vi "viewer.vi"(8 "Color Box":u32(colorbox)=5896447, 11 "Ibeo":dbl[][](array[numeric])=[[-8.194514690670069, 12.209047268904888, 0.20057577918921865, -1.2], [-7.922188195282239, 12.530063176191208, 0.1993192339962172, -1.2], [-7.848906696184014, 12.605199714224918, 0.19910980979738363, -1.2], [-8.31093082702301, 12.33609318816849, 0.3656663756006245, -0.3999999999999999], [-8.273047603432309, 12.451558326925204, 0.36524749998274675, -0.3999999999999999], [-8.066578783002836, 12.699122833174604, 0.36489843696784874, -0.3999999999999999], [-7.908452357315748, 12.841755311057485, 0.1945024774230451, -1.2], [-7.895234983174988, 12.994568657418597, 0.19219881123587584, -1.2], [-8.062522647946755, 12.859777292173597, 0.3640606857320933, -0.3999999999999999], [-7.824791817030648, 13.99344470034109, 0.17649199632335816, -1.2], [-8.063674699079533, 13.931801029401951, 0.3581964270818056, -0.3999999999999999], [-7.8135978930264125, 14.173967995680819, 0.17356005753968817, -1.2], [-8.031209860249872, 14.080843843301425, 0.35749830105200947, -0.3999999999999999], [-7.82276958407434, 14.387850587687291, 0.1697904219606839, -1.2], [-8.073152114569078, 14.335283323635828, 0.3558926111834783, -0.3999999999999999], [-7.891075140636294, 14.693334221257622, 0.1637171201945104, -1.2], [-8.111243508180511, 14.591251758204468, 0.35428692131494716, -0.3999999999999999], [-7.837216119361166, 14.82676657508684, 0.16204172660384186, -1.2], [-8.065161930030882, 14.734022733414673, 0.35365860788813064, -0.3999999999999999], [-7.8864594284729, 15.11851517851068, 0.15638727323533547, -1.2], [-8.136133319461743, 15.049896083998677, 0.35156422979874213, -0.3999999999999999], [-8.062386760128094, 15.160595778342891, 0.35121516678384407, -0.3999999999999999], [-7.9015329362479765, 15.597469450579638, 0.14780088108315914, -1.2], [-8.030734784039595, 15.565267383057458, 0.3489811634884964, -0.3999999999999999], [-7.837442171074448, 15.732479146376736, 0.14612548749249055, -1.2], [-8.048111766595339, 15.827552126486646, 0.34737547361996524, -0.3999999999999999], [-7.860387428879935, 16.012208734234335, 0.1408898825216513, -1.2], [-8.056202749080104, 16.08256925295217, 0.3458395963544137, -0.3999999999999999], [-7.87387677823714, 16.284689646223693, 0.13586370174964563, -1.2], [-7.837519828869938, 16.480818892560503, 0.13272233876714212, -1.2], [-8.06566035168659, 16.347183699638233, 0.3442339064858825, -0.3999999999999999], [-11.669869640901991, 13.268898159351348, 0.3442339064858825, -0.3999999999999999], [-11.623722029161186, 13.581091757690992, 0.34304709223522906, -0.3999999999999999], [-7.823316745669438, 16.72057446606854, 0.12853385479047075, -1.2], [-8.055641790260522, 16.587197426343405, 0.3428376544262902, -0.3999999999999999], [-8.042029216167052, 16.82800693693079, 0.3414414023666979, -0.3999999999999999], [-7.820276479008444, 16.98716777957602, 0.1237170982172986, -1.2], [-11.673363951247808, 13.989217618076957, 0.34088290154286094, -0.3999999999999999], [-11.802226900015416, 13.921712225849964, 0.34053383852796293, -0.3999999999999999], [-8.049807482572618, 17.112867929828568, 0.3396960872922075, -0.3999999999999999], [-11.712420247707064, 14.212131313250396, 0.3396262746892279, -0.3999999999999999], [-11.712185704759628, 14.402104547594199, 0.3387187108504929, -0.3999999999999999], [-11.680735996678221, 14.56510231725602, 0.33809039742367636, -0.3999999999999999], [-7.8114890300212805, 17.540707439157913, 0.1136647366732873, -1.2], [-8.018268387774892, 17.624731922838397, 0.33669414536408404, -0.3999999999999999], [-11.72577268948283, 14.805480140404125, 0.33669414536408404, -0.3999999999999999], [-7.800708178599534, 17.818889350133773, 0.10863855590128157, -1.2], [-11.710914134211848, 14.990914134211849, 0.33585639412832863, -0.3999999999999999], [-11.665658577131227, 15.1484193030316, 0.3352978933044917, -0.3999999999999999], [-8.027699153236274, 17.938916949360994, 0.33473939248065476, -0.3999999999999999], [-7.804112965736486, 18.133414204998054, 0.1027746783339416, -1.2], [-8.011648084453142, 18.061238599938417, 0.5659587335491414, 0.40000000000000013], [-8.014847599185678, 18.067193186426245, 0.7980630184613928, 1.2000000000000006], [-11.701887182530728, 15.392329358999303, 0.3339016412448994, -0.3999999999999999], [-11.18235494553231, 15.899808863285491, 0.3337620160389402, -0.3999999999999999], [-8.0322354499762, 18.254328816861292, 0.3327846395972256, -0.3999999999999999], [-11.62775268829881, 15.738382844333326, 0.3325053891853071, -0.3999999999999999], [-11.73472519046489, 15.637753162553611, 0.3325053891853071, -0.3999999999999999], [-7.802601115554845, 18.449075343828376, 0.09691080076660175, -1.2], [-8.008769879914695, 18.526556479295465, 0.33117894972869444, -0.3999999999999999], [-7.831841217452702, 18.837389870324824, 0.08937152960859324, -1.2], [-7.985685070733222, 18.808397837650894, 0.3295034472571836, -0.3999999999999999], [-7.762836832549808, 19.038628603093233, 0.08623016662608962, -1.2], [-7.998428267279901, 19.17151180169247, 0.3271996313588563, -0.3999999999999999], [-7.807112712480842, 19.4834706448484, 0.07743435027507978, -1.2], [-8.036104747242254, 19.598910858367518, 0.3244071272396717, -0.3999999999999999], [-8.021956225472685, 19.750254373746202, 0.5765004365990634, 0.40000000000000013], [-8.049686111962624, 19.992036352840987, 0.3218938735324055, -0.3999999999999999], [-7.994407959440638, 20.062524792131466, 0.578385376879513, 0.40000000000000013], [-8.040090666069212, 20.350354036833295, 0.3196598702370579, -0.3999999999999999], [-7.999678783030214, 20.45726955656002, 0.5808986305867792, 0.40000000000000013], [-8.024832769245576, 20.7097434285252, 0.31742586694171016, -0.3999999999999999], [-7.9904318259420295, 20.835113251217667, 0.5832722590880861, 0.40000000000000013], [-8.0201622485404, 21.106673826814433, 0.31491261323444397, -0.3999999999999999], [-7.995314329012896, 21.25983310220247, 0.5859949506042911, 0.40000000000000013], [-8.001177834809809, 21.48647283041383, 0.31253898473313707, -0.3999999999999999], [-7.9575040474444485, 22.048783880339585, 0.5909516454158438, 0.40000000000000013], [-8.046483670341773, 22.0329497364633, 0.308908729378197, -0.3999999999999999], [-8.025433114646795, 22.442977434942478, 0.3063256630679513, -0.3999999999999999], [-7.9802625842223485, 22.569711190455976, 0.594372462961845, 0.40000000000000013], [-8.009054805576646, 22.88184322956092, 0.30353315894876665, -0.3999999999999999], [-7.968571393744589, 23.027403979048092, 0.5973045922869888, 0.40000000000000013], [-7.990899654200996, 23.856241946520424, 0.2972500246806013, -0.3999999999999999], [-8.000898076518773, 24.152091251589102, 0.6047047282028281, 0.40000000000000013], [-8.011964114086332, 24.457778204016666, 0.29327070631076324, -0.3999999999999999], [-7.972054867346523, 24.63260748666816, 0.6077764827339311, 0.40000000000000013], [-7.988910651645925, 24.9672300085195, 0.28998951397072126, -0.3999999999999999], [-7.938790538019864, 25.123578481570966, 0.6109180498680138, 0.40000000000000013], [-7.984256066269928, 25.553256654635888, 0.2861498208068424, -0.3999999999999999], [-7.943696922487425, 25.74772056172415, 0.6150369934438111, 0.40000000000000013], [-8.005768122858095, 26.24480723490346, 0.2815421890101878, -0.3999999999999999], [-7.973645924100258, 26.477717681601202, 0.6199238756523843, 0.40000000000000013], [-7.996752928404116, 26.88147248348014, 0.2773534328314109, -0.3999999999999999], [-7.966378125571135, 27.133912528293944, 0.6242522570371204, 0.40000000000000013], [19.072594357887944, 19.847646565571097, 0.273513739667532, -0.3999999999999999], [-7.974119624650943, 27.510164161678034, 0.27323448925561356, -0.3999999999999999], [18.966327804266037, 20.047570235996055, 0.2731646766526339, -0.3999999999999999], [18.940416091600433, 20.31977342712424, 0.2720476750049601, -0.3999999999999999], [-7.966530139110388, 27.848833218611254, 0.6289995140397342, 0.40000000000000013], [19.617239241951573, 20.16420326208543, 0.6308146417172042, 0.40000000000000013], [19.470454947247852, 20.336065589851415, 0.6308146417172042, 0.40000000000000013], [-7.938090412265838, 28.130667071877102, 0.26918535828279583, -0.3999999999999999], [19.481777877437366, 20.34582205069638, 0.9928275233766126, 1.2000000000000006], [19.68969208752365, 20.225539123400168, 0.9945029169672812, 1.2000000000000006], [-7.904373212400746, 28.403162954359185, 0.6325599567916946, 0.40000000000000013], [-11.218347998608445, 29.1922777087403, 0.645754538754842, 0.40000000000000013], [-11.255655930488722, 29.279114272061154, 1.0393196955176651, 1.2000000000000006], [-7.931052931321677, 30.565756380981856, 0.2529190217885454, -0.3999999999999999], [-7.915722020860143, 30.965173285836535, 0.64973385712468, 0.40000000000000013], [19.643079014175772, 25.999680999909852, 0.6595774341448059, 0.40000000000000013], [19.678772386784143, 26.04038149087464, 1.0799479900913775, 1.2000000000000006], [19.794377409040397, 25.97301782491852, 0.23986406503135732, -0.3999999999999999], [16.951716843249166, 28.313152412727153, -0.18246108047738013, -1.2], [17.23702345210269, 28.261242886298856, -0.18497417086338291, -1.2], [17.355126239459604, 28.42991114665332, 0.2369319357062135, -0.3999999999999999], [17.500999358199543, 28.40558641198749, 1.0906286242318897, 1.2000000000000006], [17.521755060239993, 28.434955051084508, 0.6637661903235827, 0.40000000000000013], [-9.551271036081815, 33.70704072673605, 1.1140841345012495, 1.2000000000000006], [17.026214692366207, 30.91768945041584, -0.22895325261843263, -1.2], [16.947627408349614, 31.330792132214754, -0.23544540278227327, -1.2], [21.974210360871428, 29.796607180878567, 0.20970502054416343, -0.3999999999999999], [21.858954092414884, 29.892890962266808, 0.6902949794558367, 0.40000000000000013], [23.61693994019074, 29.825860936769622, 0.2020256342164057, -0.3999999999999999], [26.517784402942883, 29.636358746131258, 0.18897067745921764, -0.3999999999999999], [26.28807825554624, 29.868078255546244, 0.18897067745921764, -0.3999999999999999], [27.494195142074055, 29.89355973078797, 0.7171728316029887, 0.40000000000000013], [-9.596819805221863, 41.319124757332645, 0.17738178536460142, -0.3999999999999999], [-9.614421585529625, 42.10789864388739, 0.727993785064829, 0.40000000000000013], [-9.657997961001028, 43.03366172097774, 0.16565326806402603, -0.3999999999999999], [-9.654708582864293, 43.79505415648642, 0.7395128645564657, 0.40000000000000013], [-9.644952612918221, 44.55715817032658, 0.15532100282304295, -0.3999999999999999], [-9.649848604658922, 44.578365040432125, -0.43460781587299796, -1.2], [-9.613637000791527, 45.25325758295734, 1.3482203887971804, 1.2000000000000006], [-9.659620726679865, 45.4564764101684, 0.7508225062391634, 0.40000000000000013], [-9.631988411628107, 46.20048575995598, 0.14415098634630447, -0.3999999999999999], [-9.607672332879817, 47.92485002284773, 0.13242246904572907, -0.3999999999999999], [17.086090559334245, 45.56061718044098, 1.4035083772892427, 1.2000000000000006], [17.292711367504157, 45.540430347987886, -0.5047649224822437, -1.2], [17.52268129512945, 45.574561388711366, 1.407278012868247, 1.2000000000000006], [17.557063414189265, 45.656553436391754, 0.7696719090436596, 0.40000000000000013], [15.905718653071306, 48.76995079198919, 0.11420137966804939, -0.3999999999999999], [15.711030412050338, 48.84901591474403, 0.7858684329349304, 0.40000000000000013], [27.308705200532295, 43.3826639824295, 0.11154850075482398, -0.3999999999999999], [27.522668444206523, 43.31998672256406, 0.7889401874660336, 0.40000000000000013], [25.383882599796944, 45.09750939942709, 0.10882580923861901, -0.3999999999999999], [15.378656492958747, 49.840262152105595, -0.5751314532903231, -1.2], [15.600149970456558, 49.82844562031466, 0.7920817546001162, 0.40000000000000013], [15.416587087242455, 49.95362474886922, 0.1074993697820063, -0.3999999999999999], [25.68368027358097, 46.42446403292412, 0.09981998345424858, -0.3999999999999999], [25.383632788769415, 46.777506687909195, 0.09877279440955439, -0.3999999999999999], [-8.027847677156654, 53.1687727040271, 0.09842373139465632, -0.3999999999999999], [-8.695167719437398, 53.15994682681221, 0.80227439463514, 0.40000000000000013], [20.483247073305144, 49.77303169169489, 0.09584066508441053, -0.3999999999999999], [20.078047311320553, 49.95132385408298, 0.09584066508441053, -0.3999999999999999], [19.718193698014808, 50.23653112811276, 0.09500291384865517, -0.3999999999999999], [25.429376633443997, 47.73477995506515, 0.09283872315628705, -0.3999999999999999], [-9.338780758706811, 54.24462327975186, 0.8105122817867347, 0.40000000000000013], [16.860460258517662, 52.83196371705928, -0.6444508631042345, -1.2], [25.652365748645803, 49.03552706564198, 0.08418196038681475, -0.3999999999999999], [32.06392885145435, 45.03486562995687, 1.5521995584610773, 1.2000000000000006], [31.778479775771135, 45.41808238881591, 0.818261480717472, 0.40000000000000013], [31.77225525537603, 45.40989672895938, 1.55471264884708, 1.2000000000000006], [25.423084254782847, 49.565065245207975, 0.08173851928252823, -0.3999999999999999], [32.6300247772637, 45.011263200800904, 1.559110557022585, 1.2000000000000006], [32.69832444037635, 45.09790091043385, 0.8204256714098401, 0.40000000000000013], [25.439400701881368, 50.55981320376924, 0.075595010220322, -0.3999999999999999], [34.51917188715493, 45.11514830598214, 1.5857074302744485, 1.2000000000000006], [34.92683747694728, 44.86443385971285, 1.5871733996662833, 1.2000000000000006], [25.42149285051838, 51.52298336238443, 0.06973075157003433, -0.3999999999999999], [35.54812755297423, 44.85971643116604, 1.595550367619626, 1.2000000000000006], [34.609532792271075, 45.973543243462, 1.6007859725904654, 1.2000000000000006], [25.46718877424603, 52.64016177857301, 0.06267967866909313, -0.3999999999999999], [34.731322610921104, 46.89122723132968, 1.6173304842983174, 1.2000000000000006], [25.468059591047258, 53.70827288404634, 0.05604748138602972, -0.3999999999999999], [41.47455368343372, 42.586470182247886, 1.6470687205326844, 1.2000000000000006], [25.474515940300442, 54.8248279005798, 0.04906622108806813, -0.3999999999999999], [17.65203521232784, 58.21903070119556, 0.04780959423443509, -0.3999999999999999], [20.295637544941265, 57.39533782171512, 0.8528885317953614, 0.40000000000000013], [17.443289950392376, 58.39142219368391, 0.8528885317953614, 0.40000000000000013], [20.330615094364084, 57.487659485279245, 1.6608907176556997, 1.2000000000000006], [-7.75035495317097, 61.16042739371937, 0.04348121284969886, -0.3999999999999999], [17.389741843531517, 59.058954065737105, 0.04278308681990278, -0.3999999999999999], [25.459018306497637, 55.93626861288663, 0.04215477339308621, -0.3999999999999999], [43.67980265747188, 42.54959453739267, 0.8601490425052414, 0.40000000000000013], [43.68617582564682, 42.555282807469325, 1.680786016544889, 1.2000000000000006], [35.131445440240526, 50.67758542316679, 1.685183924720394, 1.2000000000000006], [25.54658114567024, 57.304002719404814, 0.033288572814675066, -0.3999999999999999], [35.35626866103595, 51.854440322607054, 1.7078017381944195, 1.2000000000000006], [31.93987374886766, 54.289371727955974, 1.7096865559839216, 1.2000000000000006], [32.39423109821591, 54.025674009004575, 0.8699926195253671, 0.40000000000000013], [31.951466968313056, 54.30774586871799, 0.8699926195253671, 0.40000000000000013], [32.40411221068225, 54.04103591888299, 1.710524252779256, 1.2000000000000006], [17.757709303896025, 61.10224897949335, 0.8715983093938983, 0.40000000000000013], [17.763112456640282, 61.11964997506754, 1.715341009352428, 1.2000000000000006], [35.4230011788845, 52.84401581410436, 1.7253933708964393, 1.2000000000000006], [29.290605081293037, 57.09313695219341, 0.8773229428382268, 0.40000000000000013], [40.759454288225115, 49.265171081946534, 1.7369117018322857, 1.2000000000000006], [40.82070045763014, 49.33379161726375, 0.8795569461335744, 0.40000000000000013], [30.505508525730225, 57.06601565541906, 0.8813022612080648, 0.40000000000000013], [41.460377534907316, 49.23945311745191, 1.7463357907797963, 1.2000000000000006], [31.138639213649242, 57.081515746789364, 0.8836060771063922, 0.40000000000000013], [46.014679894453145, 45.363042821123074, 1.7563881523238076, 1.2000000000000006], [31.743685463928472, 57.03846551713426, 0.8854910173868418, 0.40000000000000013], [17.31309627006752, 63.34316908027608, 1.757225849119142, 1.2000000000000006], [42.29288815694243, 49.34445773182582, 1.7597389395051446, 1.2000000000000006], [42.32831546364073, 49.38278277629349, 0.886887269446434, 0.40000000000000013], [17.88136701557938, 63.34167325680246, 1.760576636300479, 1.2000000000000006], [17.62830080143847, 63.44853765546489, -0.8612049088969791, -1.2], [26.330614951038932, 60.21786202185187, 0.012554229729729194, -0.3999999999999999], [17.65164798186575, 63.527356415664414, 0.012414604523770023, -0.3999999999999999], [47.01008426653839, 44.78828389450921, 1.763927423481816, 1.2000000000000006], [32.40222865539054, 57.07441257637522, 0.8880740836970875, 0.40000000000000013], [25.875513670239723, 60.537777650039054, 0.011856103699933118, -0.3999999999999999], [26.6293328816576, 60.21031030179518, 0.8882835215060264, 0.40000000000000013], [46.08014715978688, 46.16470846246666, 1.7687441800549881, 1.2000000000000006], [42.986510275999805, 49.28546090702975, 1.7687441800549881, 1.2000000000000006], [43.001773126855184, 49.30168579532624, 0.8896797735656188, 0.40000000000000013], [33.053289421972515, 57.08591780848661, 0.8905175248013741, 0.40000000000000013], [27.810809593833586, 60.12891297351032, 0.8913552760371295, 0.40000000000000013], [28.381044878981022, 60.03455577612013, 0.892542090287783, 0.40000000000000013], [43.74453500294738, 49.28282946195488, 1.779634238394334, 1.2000000000000006], [43.7807538462754, 49.320664159288334, 0.8935194667294976, 0.40000000000000013], [29.034172134534455, 60.094571689007886, 0.8949855313920695, 0.40000000000000013], [33.007900723397846, 58.07252925361201, 1.7888489031430108, 1.2000000000000006], [44.456936817843705, 49.220301489779224, 1.7890583273418446, 1.2000000000000006], [46.04948811909361, 47.65638847280743, 1.7896865999383451, 1.2000000000000006], [29.676539302590022, 60.120926504325595, 0.8972195346874172, 0.40000000000000013], [35.011187934883196, 57.05972422411814, 0.8977082229082745, 0.40000000000000013], [33.71496149053915, 58.15516795644601, 1.798063567891688, 1.2000000000000006], [30.345242991048533, 60.18440716399954, 0.899802600997663, 0.40000000000000013], [46.03418115539351, 48.42063740041821, 1.8005766582776908, 1.2000000000000006], [45.264883119017476, 49.24294212516751, 0.9003611018214999, 0.40000000000000013], [45.27010660401662, 49.24821139373152, 1.801414355073025, 1.2000000000000006], [35.70007347446228, 57.083426553861436, 0.9005007270274591, 0.40000000000000013], [36.43705672696408, 57.16529006773202, 0.9038517319704806, 0.40000000000000013], [46.01612590764641, 49.194998161989155, 1.81167614081587, 1.2000000000000006], [36.15966107692616, 57.7712480081585, 1.819005987775045, 1.2000000000000006], [36.6606234208242, 57.493641736840296, 1.820053108769213, 1.2000000000000006], [-8.177338024764591, 68.80742176813614, -0.009855615826727393, -0.3999999999999999], [-10.750713863357651, 68.52082411852233, 0.9104141166505646, 0.40000000000000013], [-9.61269756533645, 68.69308906088567, 1.8313620155062258, 1.2000000000000006], [-10.753468452548912, 68.53773793044842, 1.8317808639038928, 1.2000000000000006], [-9.053602299804032, 68.85243249537551, 1.8330374090968942, 1.2000000000000006], [-9.628891609205853, 68.80477743727172, 0.9111820552833403, 0.40000000000000013], [-8.48739895001441, 68.9673105066083, 1.8338751058922282, 1.2000000000000006], [-9.06342927181574, 68.92463972020676, 0.9114613056952587, 0.40000000000000013], [-7.91986828558831, 69.07728568096844, 1.8347128026875628, 1.2000000000000006], [-8.49659641301999, 69.0396084729745, 0.9117405561071772, 0.40000000000000013], [26.15903687971658, 64.66594184335025, 0.9153009988591376, 0.40000000000000013], [-7.832914886648823, 70.86207853253605, -0.02381813642265046, -0.3999999999999999], [37.4382212217352, 60.761565188583845, 1.8860217314017873, 1.2000000000000006], [18.008301688605677, 71.19770448104013, -0.03980522250498236, -0.3999999999999999], [17.521390036357968, 71.76019525864842, -0.042737351830126225, -0.3999999999999999], [24.707418244399033, 71.72519533242571, -0.057397998455845534, -0.3999999999999999], [25.4005078736632, 71.76793753964616, -0.05935275133927481, -0.3999999999999999], [29.336671765353064, 70.443559210931, 1.9836134080582308, 1.2000000000000006], [28.88493627597922, 71.01064452720468, 1.9907338308185722, 1.2000000000000006], [30.731941029775644, 70.41810854280492, 1.995131738994077, 1.2000000000000006], [31.40489903638531, 70.33595941077351, 1.9995296471695818, 1.2000000000000006], [26.800235752536192, 72.7324162677129, 0.9691265157564213, 0.40000000000000013], [33.55047955588144, 70.29052623709646, 2.0183778250646034, 1.2000000000000006], [34.2928778240623, 70.30497971984025, 2.025707672023778, 1.2000000000000006], [35.06135819063845, 70.35578374755092, 2.034084639977121, 1.2000000000000006], [36.12672785520903, 70.94427374677713, 2.0554459082581453, 1.2000000000000006], [26.78930336302148, 76.45217701832445, 2.08036738791934, 1.2000000000000006], [29.652706383178973, 76.27751778533802, 0.999494998052554, 0.40000000000000013], [-7.72067149515242, 82.05442964044114, -0.10144975093598291, -0.3999999999999999], [27.274245776186877, 81.96097957697368, 2.1924093342953, 1.2000000000000006], [19.214159085788403, 89.00726942131817, 2.2879067689634076, 1.2000000000000006], [17.67305899093741, 91.03313371450287, -0.17412467063776266, -0.3999999999999999], [17.46427591689643, 91.98294494221467, 1.0803379923029488, 0.40000000000000013], [17.492049584583196, 92.12257259861751, 2.3442418784496377, 1.2000000000000006], [18.27146462529139, 91.99460640780725, 2.3448701510461385, 1.2000000000000006], [19.813310669545274, 95.37543410709782, 1.1068667814352027, 0.40000000000000013], [20.222964373123798, 95.32650364265365, -0.20714603184712072, -0.3999999999999999], [19.820025339479447, 95.40636000171534, 2.421519407819225, 1.2000000000000006], [18.94569889723199, 101.66885444951467, -0.24868453061999202, -0.3999999999999999], [-9.368563424975157, 103.7549015464845, 1.1533619750196267, 0.40000000000000013], [-9.369510694295265, 103.76521060407805, 2.5605770758447153, 1.2000000000000006], [18.228004875953722, 102.58884093792915, -0.2540601010494224, -0.3999999999999999], [24.442869756726207, 105.86667474355525, -0.2854757723902494, -0.3999999999999999], [-35.031387821082, 106.18725494762796, 2.7230902541395654, 1.2000000000000006], [17.809329188065963, 113.70441666053826, 1.2300162130912444, 0.40000000000000013], [17.820291639345548, 113.77172863568872, 2.7917813913569764, 1.2000000000000006], [19.938978343495446, 114.5235055918648, 2.814818053228669, 1.2000000000000006], [19.94467488537491, 114.55500788114598, 1.2383937254487984, 0.40000000000000013], [28.70280154480414, 113.02061687017766, 2.8238232937785126, 1.2000000000000006], [25.84311044762948, 118.30301906682834, 1.272252837893912, 0.40000000000000013], [20.01734093753071, 120.79701085226053, 1.2813982888842415, 0.40000000000000013], [-9.050953842116883, 123.20680078502134, 1.2885191743881623, 0.40000000000000013], [17.623648546502675, 122.35625934959253, -0.3894965508298765, -0.3999999999999999], [20.472195791679972, 126.6633827282827, -0.42230847423029577, -0.3999999999999999], [30.059140721266083, 126.8845684991986, 1.3373181838709136, 0.40000000000000013], [16.88644565705622, 137.34740465454428, 1.3924701402248099, 0.40000000000000013], [18.07196214070289, 137.32244576991738, 1.3933777040635449, 0.40000000000000013], [16.90078834904581, 137.46014742528823, 3.280158623036861, 1.2000000000000006], [15.730520267912945, 137.6038382777688, 3.280158623036861, 1.2000000000000006], [18.085936509259437, 137.42512748825695, 3.2826717134228636, 1.2000000000000006], [19.26838331023052, 137.35625841032368, 1.3947739561231371, 0.40000000000000013], [19.26603226944565, 137.3400435642854, 3.284347107013532, 1.2000000000000006], [16.719599816794155, 157.46521634988588, 1.5318160957721225, 0.40000000000000013], [-32.16360629620709, 157.34134738686575, 3.74298610245905, 1.2000000000000006], [-4.233287047395968, 190.56439604133394, 4.370839850562091, 1.2000000000000006], [-2.60088182180403, 190.65288518810397, 4.372096395755093, 1.2000000000000006], [16.4593091962008, 240.95418756940387, -1.212307889547625, -0.3999999999999999], [12.548942493640824, 326.63966932367794, 7.225501104862481, 1.2000000000000006], [15.378073454756912, 326.70628428865757, 7.229480164640318, 1.2000000000000006], [-11.729159678852364, 16.75029947671913, 0.32678075574097865, -0.3999999999999999], [-7.723117815283916, 27.448861100638712, -0.07753955686176178, -1.2], [-11.021927324853205, 29.356603943350766, 1.0389008471199979, 1.2000000000000006], [23.458440241517124, 29.649829187826047, -0.28905799768366697, -1.2], [29.704831196083283, 29.61198426558694, 0.7272258464320533, 0.40000000000000013], [-9.653810416305165, 43.016219342018815, -0.4027753376502952, -1.2], [-9.934710272985127, 44.98417881897335, 1.3442413290193427, 1.2000000000000006], [-9.63663164355435, 46.22143002569017, -0.4681156876863691, -1.2], [32.10082036331907, 45.082511677761076, 0.8177727924966147, 0.40000000000000013], [41.468102990551635, 42.58040197631796, 0.8489092134255232, 0.40000000000000013], [17.978610965116705, 58.40674263873944, 0.8541451586489943, 0.40000000000000013], [22.022137738709198, 56.95827563559606, 0.04550577833610775, -0.3999999999999999], [19.087353434715492, 59.29933110279508, 0.037477328993451964, -0.3999999999999999], [17.929825616719985, 62.56644496018521, 0.01827886317405769, -0.3999999999999999], [30.64216023762698, 58.41335842741442, 0.8899590239775372, 0.40000000000000013], [27.24110596115082, 60.21764008083323, 0.890168461786476, 0.40000000000000013], [46.03222952099896, 49.21096185443662, 0.90399135717644, 0.40000000000000013], [-9.881534472363711, 68.54521759315737, -0.009646178017788498, -0.3999999999999999], [-10.181857918231847, 68.60802747621722, 1.8313620155062258, 1.2000000000000006], [-10.192941210900957, 68.68003678496166, 0.9109028048714218, 0.40000000000000013], [29.343002065002473, 68.90203680303514, 0.9513243019966193, 0.40000000000000013], [29.38269505885604, 70.5481551018741, 0.9619358176495207, 0.40000000000000013], [30.055852702381053, 70.48450653814902, 1.9905244066197385, 1.2000000000000006], [30.72540321325217, 70.40392692246942, 0.9648679469746646, 0.40000000000000013], [32.169981742450176, 70.43625718481394, 2.008325463520592, 1.2000000000000006], [32.868453417655935, 70.38480009493178, 2.013770492690265, 1.2000000000000006], [36.00280500047036, 69.32786183365276, 2.024451126830777, 1.2000000000000006], [-9.351778600655775, 81.17543484742396, 0.9965628687274102, 0.40000000000000013], [20.870192909251212, 152.99644418516132, -0.6044495554041127, -0.3999999999999999], [-5.8667771546707455, 190.54162387510743, 4.371258698959759, 1.2000000000000006], [-11.687451760065155, 14.967451760065156, 0.10821970750361448, -1.2], [-9.47437053045439, 69.77634375268677, -0.017744439963423897, -0.3999999999999999], [-35.35306578150761, 147.29305575535693, 3.5524100815205015, 1.2000000000000006], [-33.56929071697392, 157.34992056763713, 1.5496183095319243, 0.40000000000000013], [-33.56913949417454, 157.3492240776528, 3.7492688284240567, 1.2000000000000006]]) -> ()   [LabVIEW 2012]
uses:
  <vilib>/Utility/miscctls.llb/LVRGBAColorTypeDef.ctl
  <vilib>/Utility/miscctls.llb/LV3DPointTypeDef.ctl
  <vilib>/picture/3D Picture Control/NI_3D Picture Control.lvlib
panel:
  out "3D Picture":refnum<vi>(3d-picture)
  in  "Color Box 3":u32(colorbox)=5896447
  in  "Color Box 2":u32(colorbox)=5896447
  in  "Scale":cluster{"X":sgl, "Y":sgl, "Z":sgl}
  in  "Angle":sgl
  in  "Axis":cluster{"X":sgl, "Y":sgl, "Z":sgl}
  in  "Translation":cluster{"X":sgl, "Y":sgl, "Z":sgl}
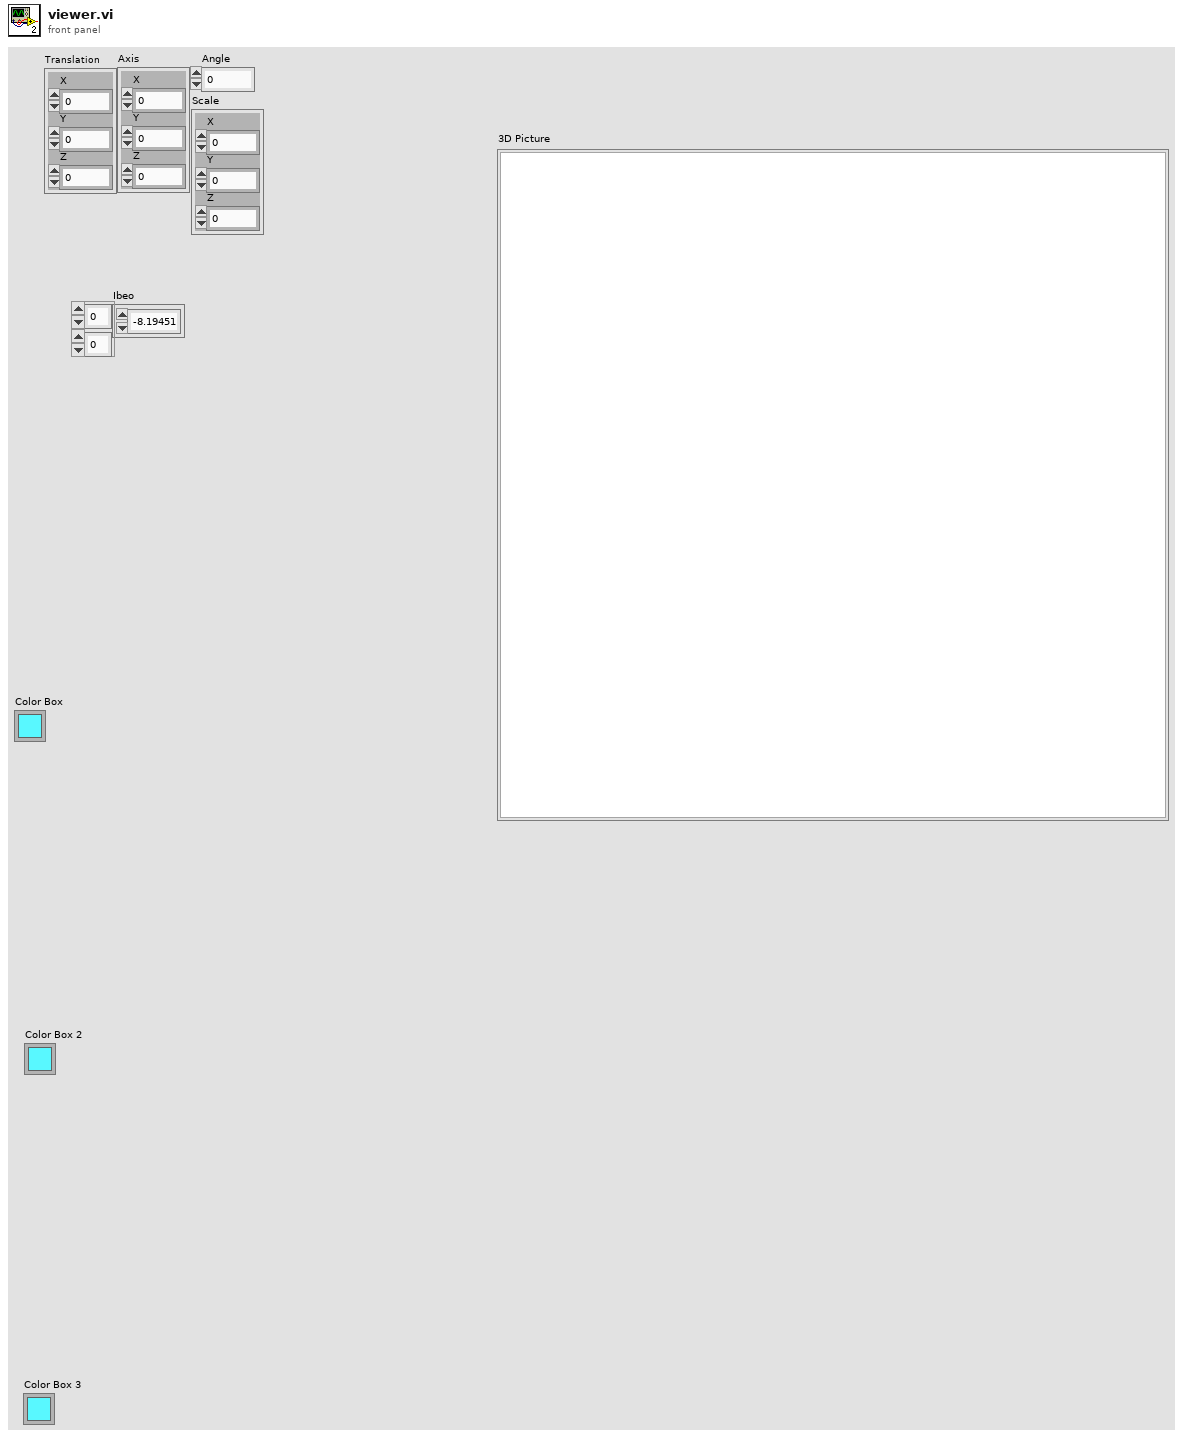
[diagram p1: front panel]
types:
  T1 = typedef "LVRGBAColorTypeDef.ctl" = cluster{"Red":sgl, "Green":sgl, "Blue":sgl, "Alpha":sgl}
  T2 = enum16{"Overall", "Per Primitive", "Per Vertex", "Binding Off"}
  T3 = enum16{"Points", "Lines", "Line Strip", "Line Loop", "Triangles", "Triangle Strip", "Triangle Fan", "Quads", "Quad Strip", "Polygon"}
  T4 = typedef "LV3DPointTypeDef.ctl" = cluster{"X":sgl, "Y":sgl, "Z":sgl}
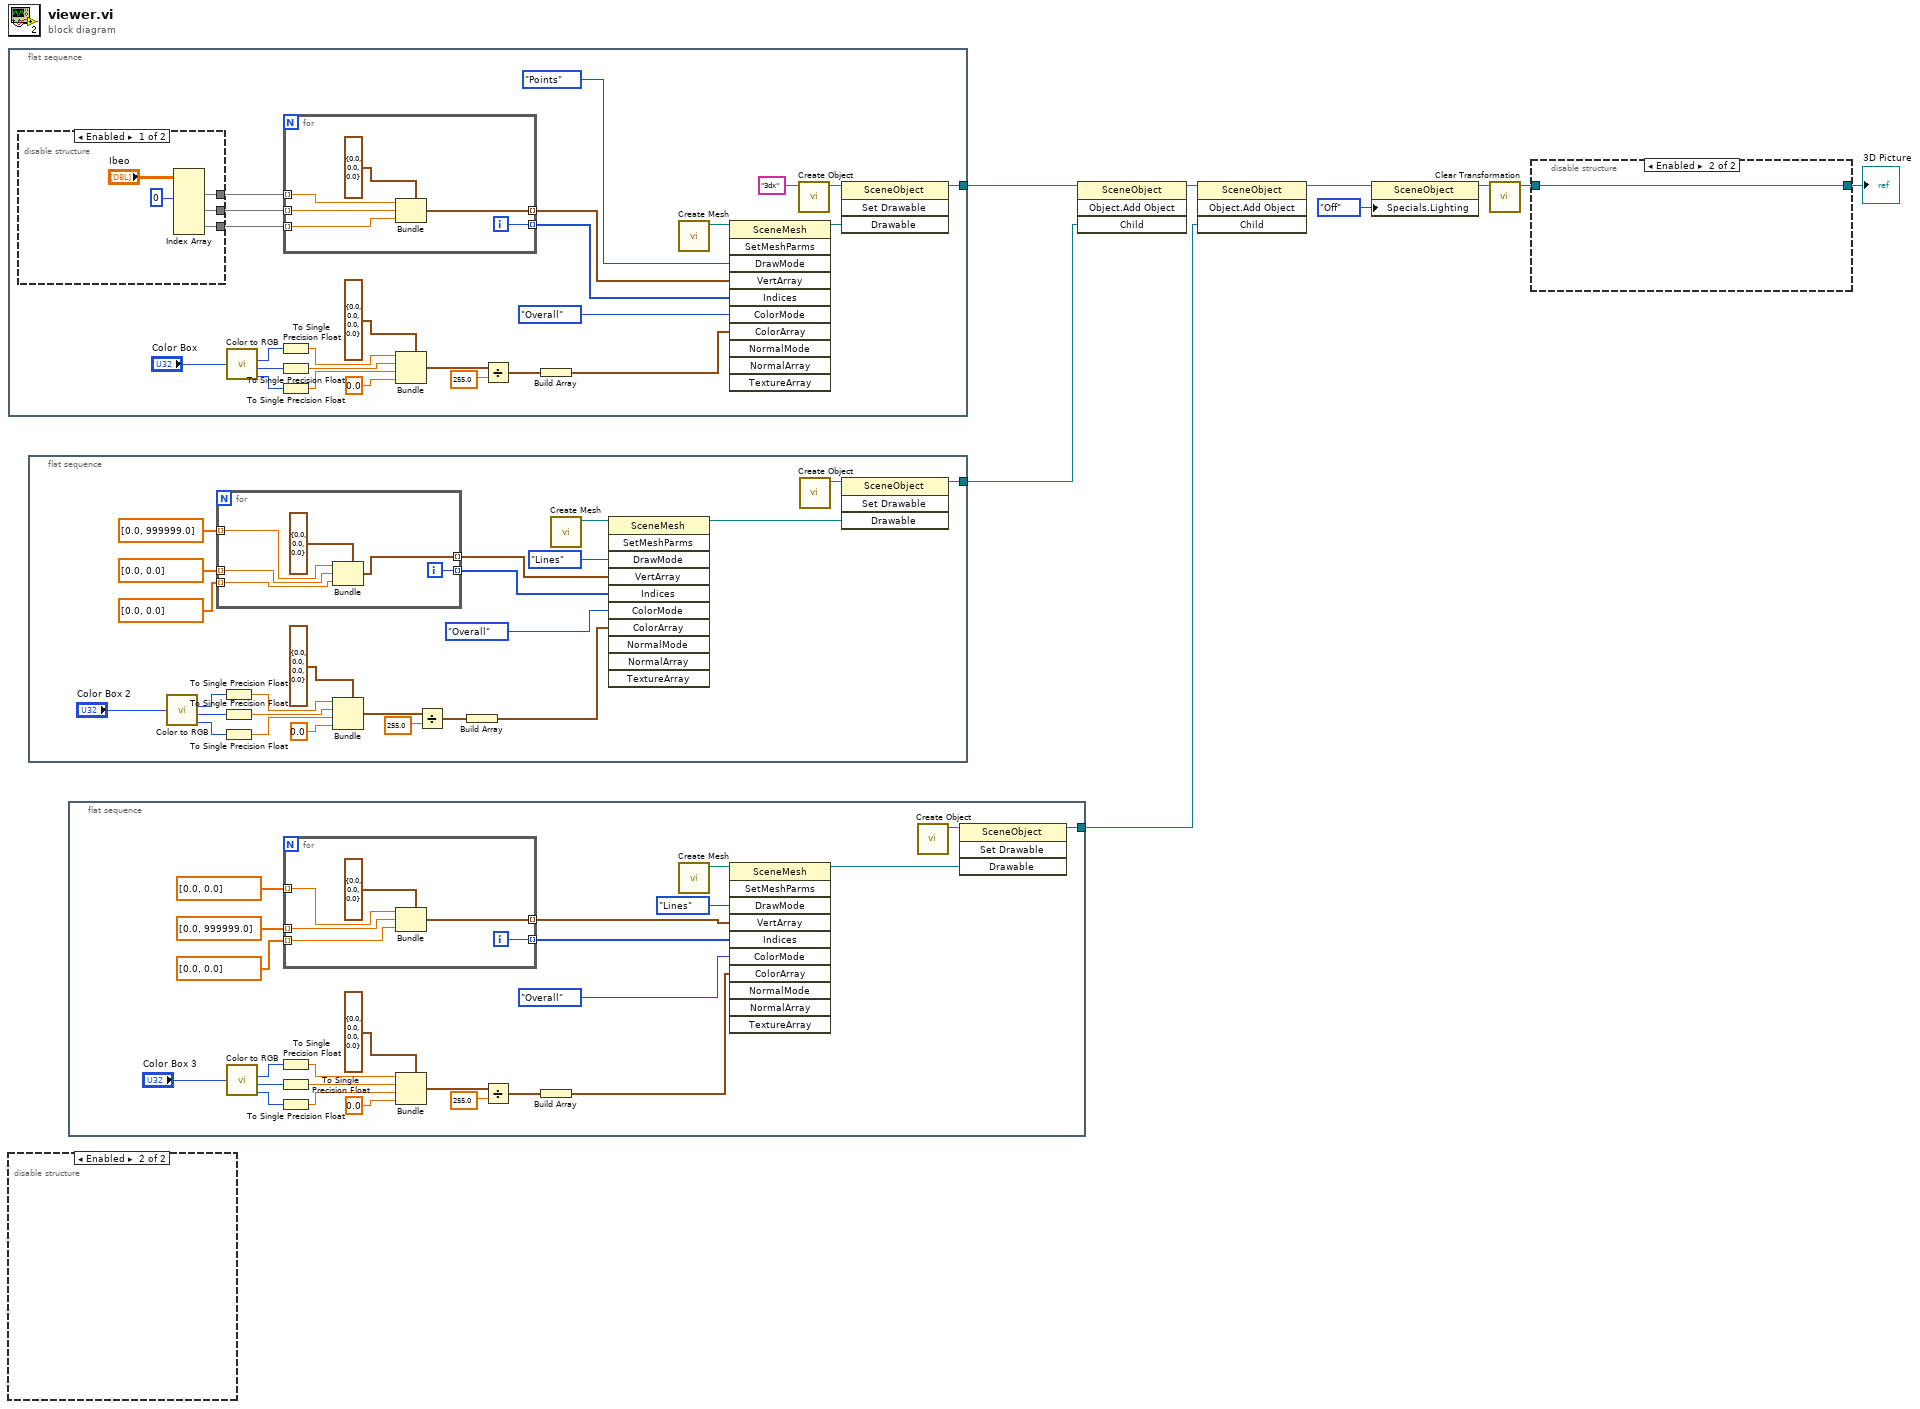
[diagram p0: block diagram]
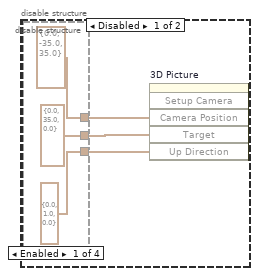
[diagram p2: hidden frame]
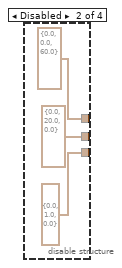
[diagram p3: hidden frame]
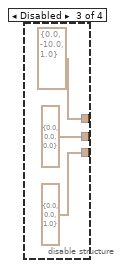
[diagram p4: hidden frame]
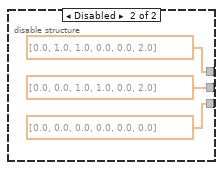
[diagram p6: hidden frame]
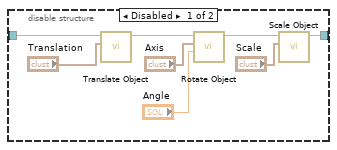
[diagram p7: hidden frame]
diagram:
  n1 = flat-sequence {
    tunnel: [w10] -> w6
    frame #0 {
      n2 = disable-structure shown="Enabled" {
        disable-tunnel: [w38 dbl[] [0.0, 0.0, 1.0, 1.0, 0.0, 2.0] ("Ibeo")] -> w32
        disable-tunnel: [w37 dbl[] [0.0, 0.0, 0.0, 0.0, 0.0, 0.0] ("Ibeo")] -> w31
        disable-tunnel: [w35 dbl[] [0.0, 1.0, 1.0, 0.0, 0.0, 2.0] ("Ibeo")] -> w11
        frame Enabled {
          n3 = Index Array(array="Ibeo", index (col) #1=0 ("disabled index (col)")) -> (element #1=w35:dbl[], element #2=w38:dbl[], element #3=w37:dbl[])  [unwired: 5 in]
        }
        frame Disabled {
        }
      }
      n4 = call <vilib>:"Color to RGB.vi"("Color"="Color Box") -> ("R"=w29:u8, "G"=w28:u8, "B"=w27:u8)  [unwired: 1 out]
      n5 = To Single Precision Float(number=w29) -> (single precision float=w25:sgl)
      n6 = To Single Precision Float(number=w28) -> (single precision float=w24:sgl)
      n7 = To Single Precision Float(number=w27) -> (single precision float=w23:sgl)
      n8 = for {
        tunnel: w11 -> [w47] mode=indexing
        tunnel: w32 -> [w46] mode=indexing
        tunnel: w31 -> [w45] mode=indexing
        tunnel: [w44] -> w17 mode=indexing
        tunnel: [w43] -> w14 mode=indexing
        i -> [w43]
        n9 = Bundle(cluster=T4 {"X"=0.0, "Y"=0.0, "Z"=0.0} ("3D Point"), "X"=w47, "Y"=w46, "Z"=w45) -> (w44:T4)
      }
      n10 = Bundle(cluster=T1 {"Red"=0.0, "Green"=0.0, "Blue"=0.0, "Alpha"=0.0} ("Color"), "Red"=w25, "Green"=w24, "Blue"=w23, "Alpha"=sgl 0.0) -> (w21:T1)
      n11 = Divide(x=w21, y=sgl 255.0) -> (x/y=w19:T1)
      n12 = Build Array(w19) -> (w15:T1[])
      n13 = call <vilib>:"Create Mesh.vi"() -> ("New Mesh Refnum"=w13:refnum<vi>)  [unwired: 10 in, 1 out]
      n14 = invoke class="SceneMesh" method="SetMeshParms"(reference=w13, "DrawMode"=T3."Points" ("Draw Mode"), "VertArray"=w17, "Indices"=w14, "ColorMode"=T2."Overall" ("Color Binding Mode"), "ColorArray"=w15) -> (reference out=w34:refnum<vi>)  [unwired: 5 in, 10 out]
      n15 = call <vilib>:"Create Object.vi"("Name"="3dx") -> ("Scene:New Object"=w12:refnum<vi>)  [unwired: 9 in, 1 out]
      n16 = invoke class="SceneObject" method="Set Drawable"(reference=w12, "Drawable"=w34) -> (reference out=w10:refnum<vi>)  [unwired: 2 in, 3 out]
    }
  }
  n17 = disable-structure shown="Enabled" {
    frame Disabled {
      n18 = disable-structure shown="Enabled" {
        disable-tunnel: [T4 {"X"=0.0, "Y"=-35.0, "Z"=35.0} ("Camera Position") T4 {"X"=0.0, "Y"=0.0, "Z"=60.0} ("Camera Position") T4 {"X"=0.0, "Y"=-10.0, "Z"=1.0} ("Camera Position") _] -> w51
        disable-tunnel: [T4 {"X"=0.0, "Y"=35.0, "Z"=0.0} ("Target") T4 {"X"=0.0, "Y"=20.0, "Z"=0.0} ("Target") T4 {"X"=0.0, "Y"=0.0, "Z"=0.0} ("Target") _] -> w50
        disable-tunnel: [T4 {"X"=0.0, "Y"=1.0, "Z"=0.0} ("Up Direction") T4 {"X"=0.0, "Y"=1.0, "Z"=0.0} ("Up Direction") T4 {"X"=0.0, "Y"=0.0, "Z"=1.0} ("Up Direction") _] -> w49
        frame Enabled {
        }
        frame Disabled {
        }
        frame Disabled {
        }
        frame Disabled {
        }
      }
      n19 = invoke on="3D Picture" class="SceneGraphDisp (strict)" method="Setup Camera"("Camera Position"=w51, "Target"=w50, "Up Direction"=w49) -> ()  [unwired: 3 in, 6 out]
    }
    frame Enabled {
    }
  }
  n20 = flat-sequence {
    tunnel: [w61] -> w5
    frame #0 {
      n21 = call <vilib>:"Color to RGB.vi"("Color"="Color Box 2") -> ("R"=w67:u8, "G"=w68:u8, "B"=w69:u8)  [unwired: 1 out]
      n22 = for {
        tunnel: dbl[] [0.0, 999999.0] ("Ibeo") -> [w89] mode=indexing
        tunnel: dbl[] [0.0, 0.0] ("Ibeo") -> [w88] mode=indexing
        tunnel: dbl[] [0.0, 0.0] ("Ibeo") -> [w87] mode=indexing
        tunnel: [w86] -> w79 mode=indexing
        tunnel: [w85] -> w82 mode=indexing
        i -> [w85]
        n23 = Bundle(cluster=T4 {"X"=0.0, "Y"=0.0, "Z"=0.0} ("3D Point"), "X"=w89, "Y"=w88, "Z"=w87) -> (w86:T4)
      }
      n24 = To Single Precision Float(number=w67) -> (single precision float=w71:sgl)
      n25 = To Single Precision Float(number=w68) -> (single precision float=w72:sgl)
      n26 = To Single Precision Float(number=w69) -> (single precision float=w73:sgl)
      n27 = Bundle(cluster=T1 {"Red"=0.0, "Green"=0.0, "Blue"=0.0, "Alpha"=0.0} ("Color"), "Red"=w71, "Green"=w72, "Blue"=w73, "Alpha"=sgl 0.0) -> (w75:T1)
      n28 = Divide(x=w75, y=sgl 255.0) -> (x/y=w77:T1)
      n29 = Build Array(w77) -> (w81:T1[])
      n30 = call <vilib>:"Create Mesh.vi"() -> ("New Mesh Refnum"=w83:refnum<vi>)  [unwired: 10 in, 1 out]
      n31 = invoke class="SceneMesh" method="SetMeshParms"(reference=w83, "DrawMode"=T3."Lines" ("Draw Mode"), "VertArray"=w79, "Indices"=w82, "ColorMode"=T2."Overall" ("Color Binding Mode"), "ColorArray"=w81) -> (reference out=w62:refnum<vi>)  [unwired: 5 in, 10 out]
      n32 = call <vilib>:"Create Object.vi"() -> ("Scene:New Object"=w63:refnum<vi>)  [unwired: 10 in, 1 out]
      n33 = invoke class="SceneObject" method="Set Drawable"(reference=w63, "Drawable"=w62) -> (reference out=w61:refnum<vi>)  [unwired: 2 in, 3 out]
    }
  }
  n34 = flat-sequence {
    tunnel: [w91] -> w2
    frame #0 {
      n35 = call <vilib>:"Color to RGB.vi"("Color"="Color Box 3") -> ("R"=w97:u8, "G"=w98:u8, "B"=w99:u8)  [unwired: 1 out]
      n36 = To Single Precision Float(number=w97) -> (single precision float=w101:sgl)
      n37 = To Single Precision Float(number=w98) -> (single precision float=w102:sgl)
      n38 = To Single Precision Float(number=w99) -> (single precision float=w103:sgl)
      n39 = for {
        tunnel: dbl[] [0.0, 0.0] ("Ibeo") -> [w119] mode=indexing
        tunnel: dbl[] [0.0, 999999.0] ("Ibeo") -> [w118] mode=indexing
        tunnel: dbl[] [0.0, 0.0] ("Ibeo") -> [w117] mode=indexing
        tunnel: [w116] -> w109 mode=indexing
        tunnel: [w115] -> w112 mode=indexing
        i -> [w115]
        n40 = Bundle(cluster=T4 {"X"=0.0, "Y"=0.0, "Z"=0.0} ("3D Point"), "X"=w119, "Y"=w118, "Z"=w117) -> (w116:T4)
      }
      n41 = Bundle(cluster=T1 {"Red"=0.0, "Green"=0.0, "Blue"=0.0, "Alpha"=0.0} ("Color"), "Red"=w101, "Green"=w102, "Blue"=w103, "Alpha"=sgl 0.0) -> (w105:T1)
      n42 = Divide(x=w105, y=sgl 255.0) -> (x/y=w107:T1)
      n43 = Build Array(w107) -> (w111:T1[])
      n44 = call <vilib>:"Create Mesh.vi"() -> ("New Mesh Refnum"=w113:refnum<vi>)  [unwired: 10 in, 1 out]
      n45 = invoke class="SceneMesh" method="SetMeshParms"(reference=w113, "DrawMode"=T3."Lines" ("Draw Mode"), "VertArray"=w109, "Indices"=w112, "ColorMode"=T2."Overall" ("Color Binding Mode"), "ColorArray"=w111) -> (reference out=w92:refnum<vi>)  [unwired: 5 in, 10 out]
      n46 = call <vilib>:"Create Object.vi"() -> ("Scene:New Object"=w93:refnum<vi>)  [unwired: 10 in, 1 out]
      n47 = invoke class="SceneObject" method="Set Drawable"(reference=w93, "Drawable"=w92) -> (reference out=w91:refnum<vi>)  [unwired: 2 in, 3 out]
    }
  }
  n48 = invoke class="SceneObject" method="Object.Add Object"(reference=w6, "Child"=w5) -> (reference out=w4:refnum<vi>)  [unwired: 2 in, 3 out]
  n49 = invoke class="SceneObject" method="Object.Add Object"(reference=w4, "Child"=w2) -> (reference out=w3:refnum<vi>)  [unwired: 2 in, 3 out]
  n50 = property class="SceneObject"(reference=w3, "Specials.Lighting"=enum16{"Inherit Value", "Off", "On"}."Off" ("Specials:Lighting")) -> (reference out=w8:refnum<vi>)  [unwired: 1 in, 1 out]
  n51 = call <vilib>:"Clear Transformation.vi"("Object Refnum In"=w8) -> ("Object Refnum Out"=w7:refnum<vi>)  [unwired: 9 in, 1 out]
  n52 = disable-structure shown="Enabled" {
    disable-tunnel: w7 -> [w122 w129]
    disable-tunnel: [w121 w129] -> w1
    frame Disabled {
      n53 = call <vilib>:"Translate Object.vi"("Translation"="Translation", "Scene.Object In"=w122) -> ("Scene.Object Out"=w128:refnum<vi>)  [unwired: 8 in, 1 out]
      n54 = call <vilib>:"Rotate Object.vi"("Angle"="Angle", "Axis"="Axis", "Scene.Object In"=w128) -> ("Scene.Object Out"=w127:refnum<vi>)  [unwired: 7 in, 1 out]
      n55 = call <vilib>:"Scale Object.vi"("Scale"="Scale", "Scene.Object In"=w127) -> ("Scene.Object Out"=w121:refnum<vi>)  [unwired: 8 in, 1 out]
    }
    frame Enabled {
    }
  }
  "3D Picture" <- w1
